vi "时间曲线生成.vi"(2 "数据":dbl[][](array[numeric]), 3 "坐标轴映射":T2, 4 "曲线设置":T3) -> (0 "曲线属性":T1[](array[typedef]), 1 "曲线":cluster{"数据":dbl[], "数据":dbl[]}[](array[cluster]))   [LabVIEW 2021]
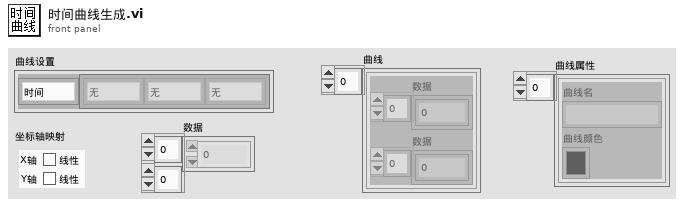
[diagram p1: front panel]
types:
  T1 = typedef "曲线属性.ctl" = cluster{"曲线名":string, "曲线颜色":u32}
  T2 = typedef "坐标轴映射.ctl" = cluster{"X轴":bool, "Y轴":bool}
  T3 = typedef "曲线设置.ctl" = cluster{"X轴数据选择":enum16{"时间", "设置电压", "读取电流", "读取电压"}, "Y轴组":enum16{"时间", "设置电压", "读取电流", "读取电压", "无"}[]}
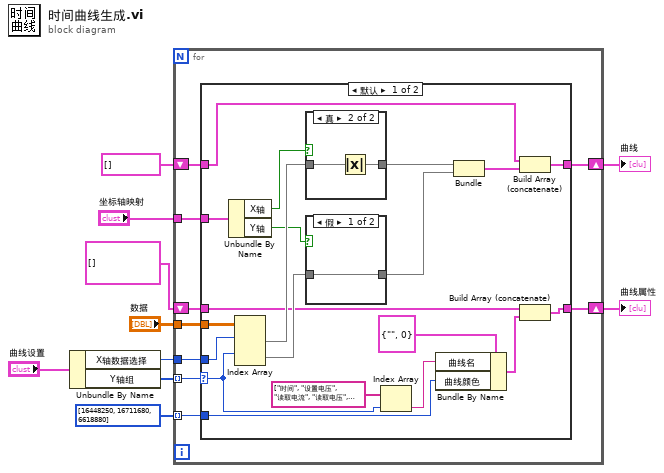
[diagram p0: block diagram]
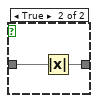
[diagram p2: hidden frame]
diagram:
  n1 = Unbundle By Name("曲线设置") -> ("X轴数据选择"=w6:enum16{"时间", "设置电压", "读取电流", "读取电压"}, "Y轴组"=w7:enum16{"时间", "设置电压", "读取电流", "读取电压", "无"}[])
  n2 = for {
    tunnel: "数据" -> [w19]
    tunnel: w6 -> [w18]
    tunnel: w7 -> [w15] mode=indexing
    shift-right: [w17] -> w9
    shift-left: cluster{"数据":dbl[], "数据":dbl[]}[] [] -> [w16]
    tunnel: "坐标轴映射" -> [w14]
    tunnel: u32[] [16448250, 16711680, 6618880] -> [w13] mode=indexing
    shift-right: [w12] -> w1
    shift-left: T1[] [] -> [w11]
    n3 = case shown="默认" w15 {
      selector: w15 -> [w23 _]
      tunnel: w19 -> [w39 _]
      tunnel: w18 -> [w38 _]
      tunnel: [w34 w47] -> w17
      tunnel: w16 -> [w33 w47]
      tunnel: w14 -> [w32 _]
      tunnel: w13 -> [w24 _]
      tunnel: [w21 w46] -> w12
      tunnel: w11 -> [w20 w46]
      frame Default {
        n4 = Unbundle By Name(w32) -> ("X轴"=w29:bool, "Y轴"=w28:bool)
        n5 = Index Array(array=w39, index (row) #1=w38, index (row) #2=w23) -> (element #1=w37:dbl[], element #2=w36:dbl[])  [unwired: 2 in]
        n6 = case shown="真" w29 {
          tunnel: w37 -> [w43 w45]
          tunnel: [w43 w44] -> w31
          frame False {
          }
          frame True {
            n7 = Absolute Value(x=w45) -> (abs(x)=w44:dbl[])
          }
        }
        n8 = case shown="假" w28 {
          tunnel: w36 -> [w40 w42]
          tunnel: [w40 w41] -> w30
          frame False {
          }
          frame True {
            n9 = Absolute Value(x=w42) -> (abs(x)=w41:dbl[])
          }
        }
        n10 = Index Array(array=string[] ["时间", "设置电压", "读取电流", "读取电压", "无"] ("字符串[]"), index=w23) -> (element=w27:string)
        n11 = Bundle By Name(cluster=T1 {"曲线名"="", "曲线颜色"=0} ("曲线属性"), "曲线名"=w27, "曲线颜色"=w24) -> (w22:T1)
        n12 = Bundle("数据"=w31, "数据"=w30) -> (w35:cluster{"数据":dbl[], "数据":dbl[]})  [unwired: 1 in]
        n13 = Build Array (concatenate)(w33, w35) -> (w34:cluster{"数据":dbl[], "数据":dbl[]}[])
        n14 = Build Array (concatenate)(w20, w22) -> (w21:T1[])
      }
      frame "无" {
      }
    }
  }
  "曲线" <- w9
  "曲线属性" <- w1
